vi "Create.vi"() -> (7 "Config Updater Identity":refnum<class "Config Updater Identity.lvclass">)   [LabVIEW 2020, in "VolatusGUI.lvlib" / "Config Updater Identity.lvclass"]
uses:
  Config Updater Identity.lvclass
  Config Updater Identity.lvclass/Config Updater Identity.ctl
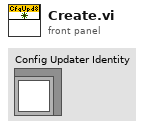
[diagram p1: front panel]
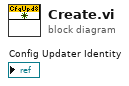
[diagram p0: block diagram]
diagram:
